vi "Create.vi"(8 "error in (no error)":errorcluster, 11 "ClientBase in":refnum<class "ClientBase.lvclass">) -> (0 "error out":errorcluster, 3 "ClientBase out":refnum<class "ClientBase.lvclass">)   [LabVIEW 2020, in "ClientBaseLib.lvlib" / "ClientBase.lvclass"]
uses:
  ClientBase.lvclass
  ClientBase.lvclass/ClientBase.ctl
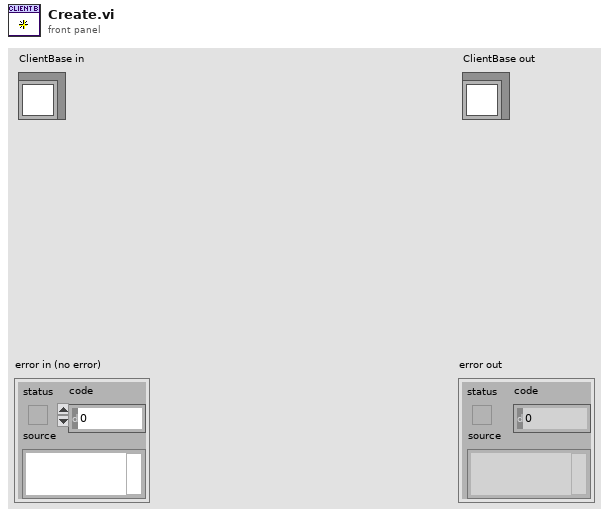
[diagram p1: front panel]
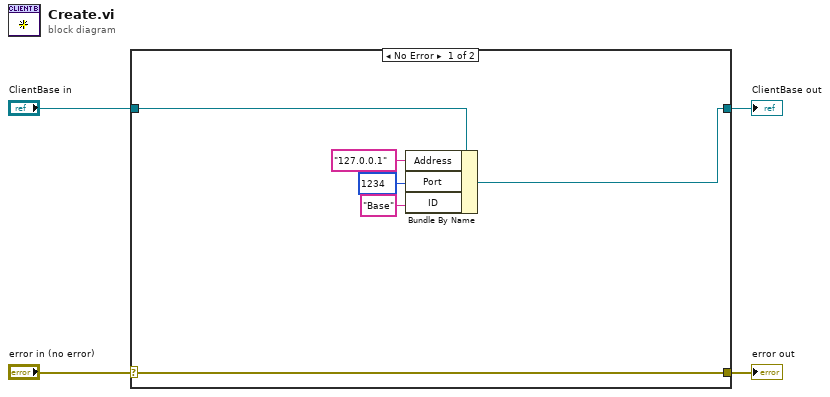
[diagram p0: block diagram]
diagram:
  n1 = case shown="No Error" "error in (no error)" {
    selector: "error in (no error)" -> [w10 w12]
    tunnel: [w10 w12] -> w3
    tunnel: [w8 w11] -> w1
    tunnel: "ClientBase in" -> [w9 w11]
    frame No Error {
      n2 = Bundle By Name(cluster=w9, "Address"="127.0.0.1", "Port"=u16 1234, "ID"="Base") -> (w8:refnum<class "ClientBase.lvclass">)
    }
    frame Error {
    }
  }
  "error out" <- w3
  "ClientBase out" <- w1
